vi "Serial,_T.O._and_Term._tl.vi"(2 "Write String":string, 3 "Terminator":string, 4 "Timeout":dbl=nan format="%.2f") -> (6 "Serial Error":bool, 7 "Read":string, 9 "T.O.":bool)   [LabVIEW 2010]
doc: "The Serial Communication VI performs bidirectional communication with a port. It initializes the port, writes a string to the port, and performs a read with timeout. The Read with Timeout will wait until a terminating character is received or the time limit is up, whichever comes first.\nThe initialisation parameters, terminating character, and timeout, are all set in the Serial Setup Global."
uses:
  Serial_Setup_tl.glob.vi
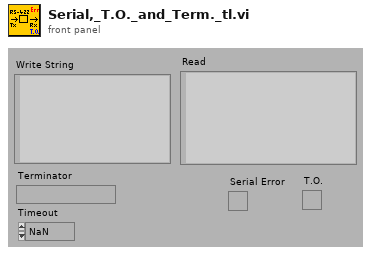
[diagram p1: front panel]
types:
  T1 = cluster{"input XON/XOFF":bool, "input HW Handshake":bool, "input alt HW HShk":bool, "output XON/XOFF":bool, "output HW Handshake":bool, "output alt HW HShk":bool, "XOFF byte ":u8, "XON byte":u8, "parity error byte":u16}
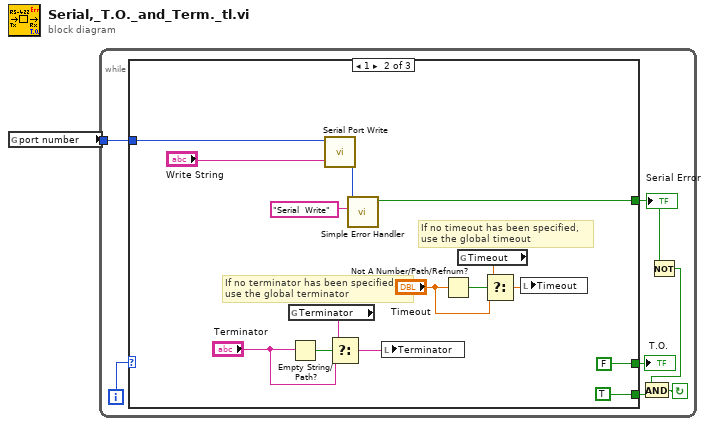
[diagram p0: block diagram]
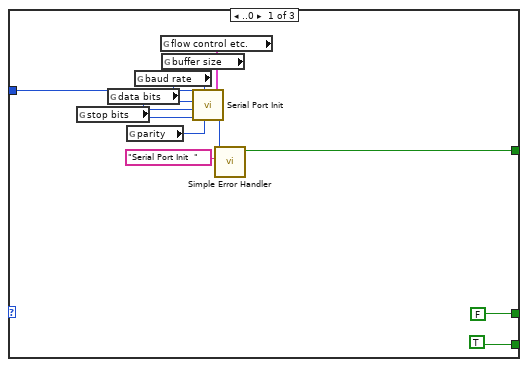
[diagram p2: hidden frame]
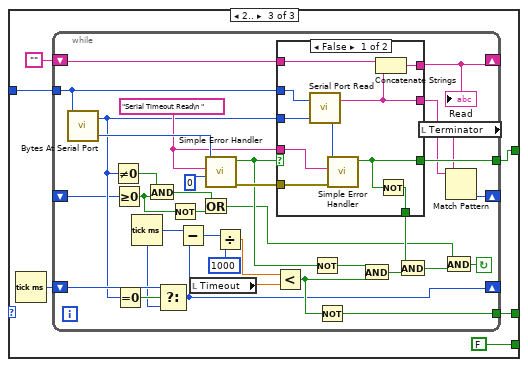
[diagram p3: hidden frame]
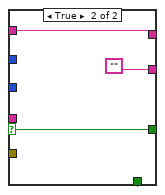
[diagram p4: hidden frame]
diagram:
  n1 = global read "Serial_Setup_tl.glob.vi" "port number"() -> (w1:i32)
  n2 = while {
    tunnel: w1 -> [w2]
    i -> [w8]
    stop <- w5 continue-if-true
    n3 = case shown="1" w8 {
      tunnel: [FALSE FALSE w39] -> w7
      tunnel: [w18 w29 w38] -> w6
      tunnel: [TRUE TRUE FALSE] -> w3
      tunnel: w2 -> [w15 w31 w36]
      frame ..0 {
        n4 = global read "Serial_Setup_tl.glob.vi" "stop bits"() -> (w13:u16)
        n5 = global read "Serial_Setup_tl.glob.vi" "data bits"() -> (w12:u16)
        n6 = global read "Serial_Setup_tl.glob.vi" "parity"() -> (w14:u16)
        n7 = global read "Serial_Setup_tl.glob.vi" "baud rate"() -> (w11:u16)
        n8 = global read "Serial_Setup_tl.glob.vi" "flow control etc."() -> (w9:T1)
        n9 = global read "Serial_Setup_tl.glob.vi" "buffer size"() -> (w10:u16)
        n10 = call <vilib>:"Serial Port Init.vi"("flow control etc."=w9, "parity"=w14, "buffer size"=w10, "stop bits"=w13, "data bits"=w12, "baud rate"=w11, "port number"=w15) -> ("error code"=w19:i32)
        n11 = call <vilib>:"Simple Error Handler.vi"("error code (no error:0)"=w19, "error source (\" \")"="Serial Port Init  ") -> ("error?"=w18:bool)  [unwired: 2 in, 5 out]
      }
      frame 1 {
        # "If no timeout has been specified,\nuse the global timeout"
        # "If no terminator has been specified,\nuse the global terminator"
        n12 = global read "Serial_Setup_tl.glob.vi" "Terminator"() -> (w27:string)
        n13 = Empty String/Path?(string/path="Terminator") -> (empty?=w28:bool)
        n14 = call <vilib>:"Serial Port Write.vi"("string to write"="Write String", "port number"=w31) -> ("error code"=w34:i32)
        n15 = Select(t=w27, s=w28, f="Terminator") -> (s? t:f=w25:string)
        n16 = call <vilib>:"Simple Error Handler.vi"("error code (no error:0)"=w34, "error source (\" \")"="Serial  Write") -> ("error?"=w29:bool)  [unwired: 2 in, 5 out]
        n17 = local write "Terminator"(w25) -> ()
        n18 = Not A Number/Path/Refnum?(number/path/refnum="Timeout") -> (NaN/Path/Refnum?=w23:bool)
        n19 = global read "Serial_Setup_tl.glob.vi" "Timeout"() -> (w24:dbl)
        n20 = Select(t=w24, s=w23, f="Timeout") -> (s? t:f=w22:dbl)
        n21 = local write "Timeout"(w22) -> ()
      }
      frame 2.. {
        n22 = Tick Count (ms)() -> (millisecond timer value=w40:u32)
        n23 = while {
          shift-left: _ -> [w42]
          shift-right: [w48] -> _
          shift-left: w40 -> [w60]
          shift-right: [w56] -> _
          shift-left: "" -> [w65]
          shift-right: [w53] -> _
          tunnel: [w72] -> w39
          tunnel: [w73] -> w38
          tunnel: w36 -> [w71]
          stop <- w61 continue-if-true
          w54 = "Serial Timeout Read\n "
          n24 = call <vilib>:"Bytes At Serial Port.vi"("port number"=w71) -> ("byte count"=w50:u32, "error code"=w57:i32)
          n25 = Not Equal To 0?(x=w50) -> (x != 0?=w49:bool)
          n26 = Greater Or Equal To 0?(x=w42) -> (x >= 0?=w44:bool)
          n27 = Equal To 0?(x=w50) -> (x = 0?=w59:bool)
          n28 = Tick Count (ms)() -> (millisecond timer value=w58:u32)
          n29 = And(x=w49, y=w44) -> (x .and. y?=w46:bool)
          n30 = Select(t=w60, s=w59, f=w58) -> (s? t:f=w56:u32)
          n31 = Not(x=w44) -> (.not. x?=w45:bool)
          n32 = Subtract(x=w58, y=w56) -> (x-y=w74:u32)
          n33 = local read "Timeout"() -> (w43:dbl)
          n34 = Or(x=w46, y=w45) -> (x .or. y?=w47:bool)
          n35 = call <vilib>:"Simple Error Handler.vi"("error code (no error:0)"=w57, "error source (\" \")"=w54, "type of dialog (OK msg:1)"=0) -> ("error?"=w64:bool, "error out"=w70:errorcluster)  [unwired: 1 in, 4 out]
          n36 = Divide(x=w74, y=u32 1000) -> (x/y=w55:dbl)
          n37 = Less?(x=w55, y=w43) -> (x < y?=w67:bool)
          n38 = case shown="False" w64 {
            selector: w64 -> [_ w87]
            tunnel: w71 -> [w83 _]
            tunnel: w50 -> [w85 _]
            tunnel: [w78 w87] -> w73
            tunnel: w70 -> [w82 _]
            tunnel: [w77 FALSE] -> w63
            tunnel: [w80 w88] -> w53
            tunnel: w65 -> [w79 w88]
            tunnel: w54 -> [w81 _]
            tunnel: [w76 ""] -> w51
            frame False {
              n39 = call <vilib>:"Serial Port Read.vi"("requested byte count"=w85, "port number"=w83) -> ("error code"=w84:i32, "string read"=w76:string)
              n40 = call <vilib>:"Simple Error Handler.vi"("error code (no error:0)"=w84, "error source (\" \")"=w81, "error in (no error)"=w82) -> ("error?"=w78:bool)  [unwired: 1 in, 5 out]
              n41 = Concatenate Strings(w79, w76) -> (w80:string)
              n42 = Not(x=w78) -> (.not. x?=w77:bool)
            }
            frame True {
            }
          }
          "Read" <- w53
          n43 = Not(x=w64) -> (.not. x?=w68:bool)
          n44 = Not(x=w67) -> (.not. x?=w72:bool)
          n45 = And(x=w68, y=w67) -> (x .and. y?=w66:bool)
          n46 = And(x=w63, y=w66) -> (x .and. y?=w62:bool)
          n47 = local read "Terminator"() -> (w52:string)
          n48 = And(x=w47, y=w62) -> (x .and. y?=w61:bool)
          n49 = Match Pattern(string=w51, regular expression=w52) -> (offset past match=w48:i32)  [unwired: 4 out]
        }
      }
    }
    "T.O." <- w7
    "Serial Error" <- w6
    n50 = Not(x=w6) -> (.not. x?=w4:bool)
    n51 = And(x=w4, y=w3) -> (x .and. y?=w5:bool)
  }
